vi "Error 7001.vi"(8 "error in (no error)":errorcluster, 10 "Build type in":string) -> (0 "error out":errorcluster)   [LabVIEW 2019, in "LVLIBP CD XML Updater.lvlib"]
uses:
  LVLIBP CD XML Updater.lvlib
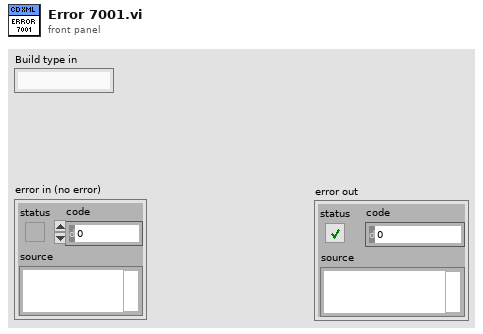
[diagram p1: front panel]
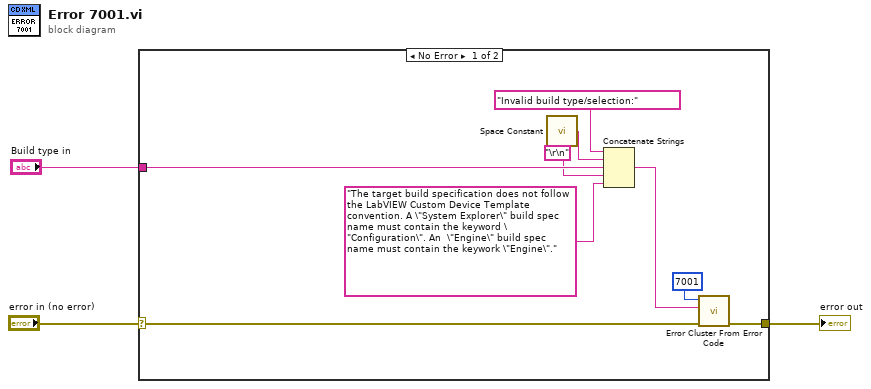
[diagram p0: block diagram]
diagram:
  n1 = case shown="No Error" "error in (no error)" {
    selector: "error in (no error)" -> [w12 w13]
    tunnel: [w11 w13] -> w2
    tunnel: "Build type in" -> [w8 _]
    frame No Error {
      n2 = call <vilib>:"Space Constant.vi"() -> ("String"=w4:string)
      n3 = Concatenate Strings("Invalid build type/selection:" ("error message (\"\")"), w4, w8, "\r\n", "The target build specification does not follow the LabVIEW Custom Device Template convention. A \"System Explorer\" build spec name must contain the keyword \"Configuration\". An  \"Engine\" build spec name must contain the keywork \"Engine\"." ("string")) -> (w6:string)
      n4 = call <vilib>:"Error Cluster From Error Code.vi"("error in (no error)"=w12, "error message (\"\")"=w6, "error code (0)"=7001) -> ("error out"=w11:errorcluster)  [unwired: 6 in]
    }
    frame Error {
    }
  }
  "error out" <- w2
